vi "Visualize alignment on RGB image.vi"(8 "error in (no error)":errorcluster, 11 "Retiga in":refnum<class "Retiga.lvclass">) -> (0 "error out":errorcluster, 3 "Retiga out":refnum<class "Retiga.lvclass">)   [LabVIEW 2012, in "Retiga.lvclass"]
uses:
  Retiga.lvclass
  Retiga.lvclass/Retiga.ctl
  <vilib>/vision/NI_Vision_Development_Module.lvlib
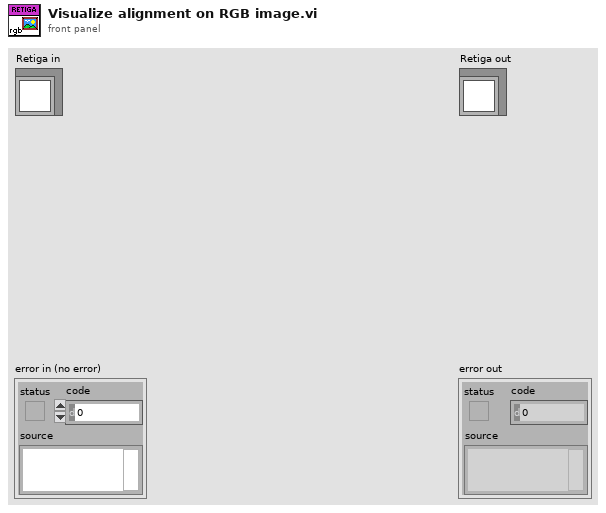
[diagram p1: front panel]
types:
  T1 = typedef "IMAQ Image.ctl" = refnum<image>
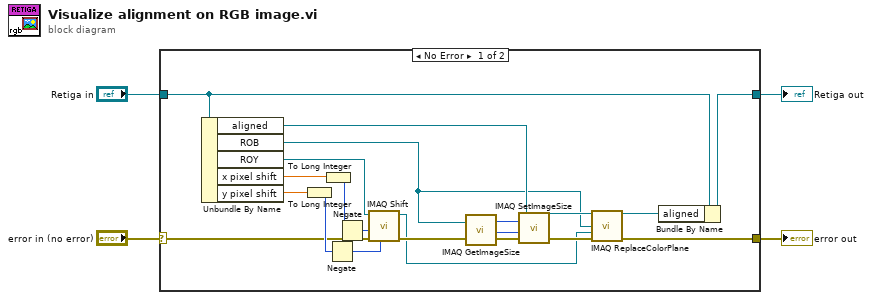
[diagram p0: block diagram]
diagram:
  n1 = case shown="No Error" "error in (no error)" {
    selector: "error in (no error)" -> [w7 w27]
    tunnel: [w6 w27] -> w3
    tunnel: [w8 w26] -> w1
    tunnel: "Retiga in" -> [w9 w26]
    frame No Error {
      n2 = Unbundle By Name(w9) -> ("aligned"=w17:T1, "ROB"=w15:T1, "ROY"=w21:T1, "x pixel shift"=w25:dbl, "y pixel shift"=w23:dbl)
      n3 = To Long Integer(number=w23) -> (32bit integer=w22:i32)
      n4 = To Long Integer(number=w25) -> (32bit integer=w24:i32)
      n5 = Negate(x=w22) -> (-x=w18:i32)
      n6 = Negate(x=w24) -> (-x=w19:i32)
      n7 = call "IMAQ Shift"("YOffset"=w18, "error in (no error)"=w7, "XOffset"=w19, "Image Src"=w21) -> ("error out"=w11:errorcluster, "Image Dst Out"=w5:T1)  [unwired: 6 in]
      n8 = call "IMAQ GetImageSize"("Image"=w15, "error in (no error)"=w11) -> ("Y Resolution"=w13:i32, "X Resolution"=w14:i32, "error out"=w12:errorcluster)  [unwired: 2 in]
      n9 = call "IMAQ SetImageSize"("error in (no error)"=w12, "Y Resolution"=w13, "X Resolution"=w14, "Image"=w17) -> ("error out"=w10:errorcluster, "Image Out"=w16:T1)  [unwired: 1 in]
      n10 = call "IMAQ ReplaceColorPlane"("Image Src"=w16, "Red or Hue Plane"=w15, "Green or Sat Plane"=w5, "error in (no error)"=w10) -> ("Image Dst Out"=w20:T1, "error out"=w6:errorcluster)  [unwired: 10 in]
      n11 = Bundle By Name(cluster=w9, "aligned"=w20) -> (w8:refnum<class "Retiga.lvclass">)
    }
    frame Error {
    }
  }
  "error out" <- w3
  "Retiga out" <- w1
